vi "User Access Level FGV Unit Test.vi"() -> ()   [LabVIEW 2017]
uses:
  User Level Cmd.ctl
panel:
  in  "Access Secure Area":bool
  out "Error Out":errorcluster
  in  "Error In":errorcluster
  in  "Current User":string
  in  "Set User Access Level":bool
  in  "stop":bool
  # "1.  Set access level for current user."
  # "2.  Test access level by verifying the appropriate dialog message."
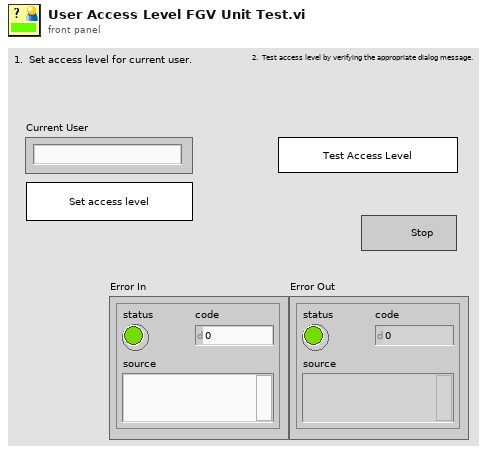
[diagram p1: front panel]
types:
  T1 = typedef "User Level Cmd.ctl" = enum16{"Read User Access Level File", "Set Current User", "Get User Access Level"}
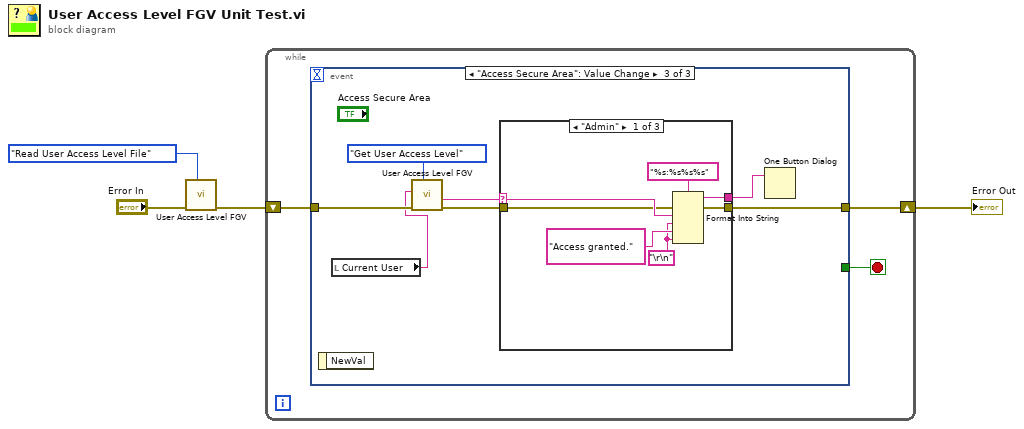
[diagram p0: block diagram]
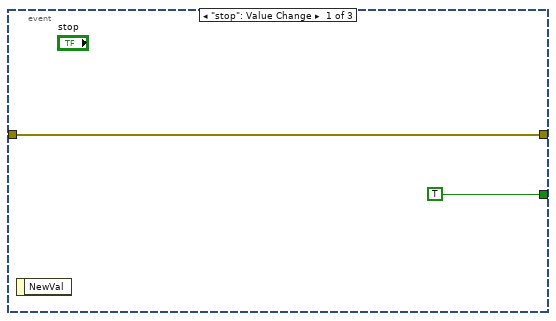
[diagram p2: hidden frame]
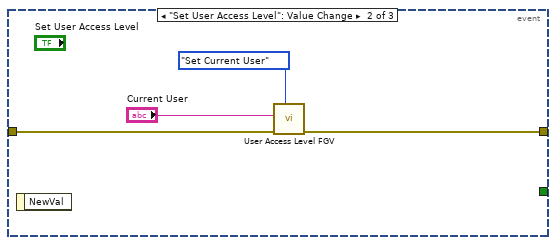
[diagram p3: hidden frame]
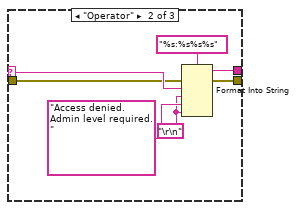
[diagram p4: hidden frame]
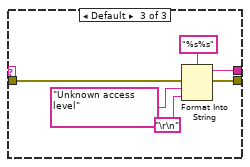
[diagram p5: hidden frame]
diagram:
  n1 = call "User Access Level FGV.vi"("User Access Level Cmd"=User_Level_Cmd."Read User Access Level File", "Error In"="Error In") -> ("Error Out"=w4:errorcluster)  [unwired: 8 in, 1 out]
  n2 = while {
    shift-right: [w5] -> w2
    shift-left: w4 -> [w6]
    stop <- w7 stop-if-true
    n3 = event shown="[2] \"Access Secure Area\": Value Change" {
      selector: _ -> [_ _ _]
      dyn-events: _ -> [_ _ _]
      timeout: _ -> [_ _ _]
      tunnel: [TRUE ("stop") _ _] -> w7
      tunnel: w6 -> [w8 w13 w20]
      tunnel: [w8 w11 w19] -> w5
      event "stop": Value Change {
        n4 = event-data() -> ()  [unwired: 1 in, 1 out]
      }
      event "Set User Access Level": Value Change {
        n5 = event-data() -> ()  [unwired: 1 in, 1 out]
        n6 = call "User Access Level FGV.vi"("User Access Level Cmd"=User_Level_Cmd."Set Current User", "Error In"=w13, "User Name"="Current User") -> ("Error Out"=w11:errorcluster)  [unwired: 7 in, 1 out]
      }
      event "Access Secure Area": Value Change {
        n7 = event-data() -> ()  [unwired: 1 in, 1 out]
        n8 = local read "Current User"() -> (w14:string)
        n9 = call "User Access Level FGV.vi"("User Access Level Cmd"=User_Level_Cmd."Get User Access Level", "Error In"=w20, "User Name"=w14) -> ("Error Out"=w18:errorcluster, "User Level"=w17:string)  [unwired: 7 in]
        n10 = case shown="\"Admin\"" w17 {
          selector: w17 -> [w27 w34 _]
          tunnel: [w25 w32 w39] -> w19
          tunnel: w18 -> [w26 w33 w40]
          tunnel: [w21 w28 w37] -> w16
          frame "Admin" {
            w23 = "\r\n"
            n11 = Format Into String(format string="%s:%s%s%s", error in=w26, w27, w23, "Access granted." ("message"), w23) -> (resulting string=w21:string, error out=w25:errorcluster)  [unwired: 1 in]
          }
          frame "Operator" {
            w30 = "\r\n"
            n12 = Format Into String(format string="%s:%s%s%s", error in=w33, w34, w30, "Access denied.  Admin level required." ("message"), w30) -> (resulting string=w28:string, error out=w32:errorcluster)  [unwired: 1 in]
          }
          frame Default {
            n13 = Format Into String(format string="%s%s", error in=w40, "Unknown access level" ("message"), "\r\n") -> (resulting string=w37:string, error out=w39:errorcluster)  [unwired: 1 in]
          }
        }
        n14 = One Button Dialog(message=w16) -> ()  [unwired: 1 in, 1 out]
      }
    }
  }
  "Error Out" <- w2
